vi "Get WideChar Length.vi"(1 "ASCII string":string caption="ASCII字符串") -> (0 "Byte Length":i32)   [LabVIEW 2012]
doc: "This VI converts an ASCII string to a unicode string."
uses:
  kernel32.dll
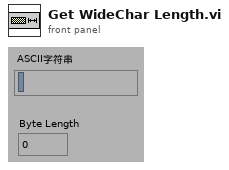
[diagram p1: front panel]
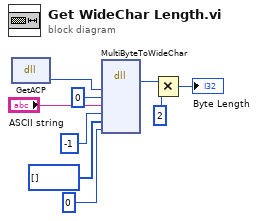
[diagram p0: block diagram]
diagram:
  n1 = dll-call lib="kernel32.dll" fn="GetACP" label="GetACP()"() -> (w9:u32)  [unwired: 3 in, 2 out]
  n2 = dll-call lib="kernel32.dll" fn="MultiByteToWideChar"("codePage"=w9, "dwFlags"=u32 0, "lpCStr"="ASCII string", "nChars"=-1, "lpWStr"=u8[] [], "nWStr"=0) -> (w3:i32)  [unwired: 9 in, 2 out]
  n3 = Multiply(x=w3, y=2) -> (x*y=→"Byte Length":i32)
